vi "Write.vi"(8 "error in (no error)":errorcluster, 9 "timeout ms (5000)":i32=5000, 10 "Bytes to write":u8[](array[numeric]), 11 "dotNET SSL Socket in":refnum<class "dotNET SSL Socket.lvclass">) -> (0 "error out":errorcluster, 2 "bytes written":i32, 3 "dotNET SSL Socket out":refnum<class "dotNET SSL Socket.lvclass">)   [LabVIEW 2013, in "dotNET SSL Socket.lvlib" / "dotNET SSL Socket.lvclass"]
doc: "Writes data to the socket.\nWebSockets 2.0.0.30\nSam Sharp - MediaMongrels Ltd\nCopyright (c) 2019, MediaMongrels Ltd"
uses:
  dotNET SSL Socket.lvclass
  dotNET SSL Socket.lvclass/dotNET SSL Socket.ctl
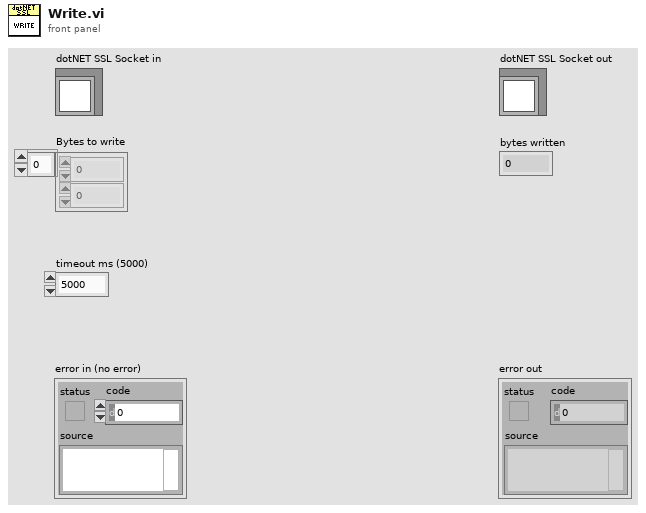
[diagram p1: front panel]
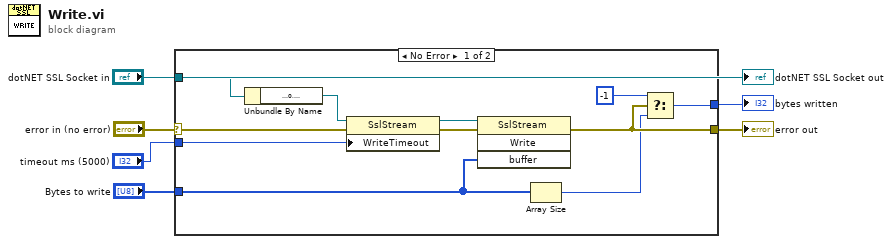
[diagram p0: block diagram]
diagram:
  n1 = case shown="No Error" "error in (no error)" {
    selector: "error in (no error)" -> [w7 w18]
    tunnel: "dotNET SSL Socket in" -> [w16 _]
    tunnel: "timeout ms (5000)" -> [w15 _]
    tunnel: [w12 w18] -> w4
    tunnel: [w11 _] -> w3
    tunnel: "Bytes to write" -> [w10 _]
    frame No Error {
      n2 = Unbundle By Name(w16) -> ("SSLStream"=w17:refnum<k24>)
      n3 = property class="SslStream"(reference=w17, error in=w7, "WriteTimeout"=w15) -> (reference out=w14:refnum<k24>, error out=w13:errorcluster)
      n4 = invoke class="SslStream" method="Write"(reference=w14, error in=w13, "buffer"=w10) -> (error out=w12:errorcluster)  [unwired: 1 in, 3 out]
      n5 = Array Size(array=w10) -> (size(s)=w9:i32)
      n6 = Select(t=-1, s=w12, f=w9) -> (s? t:f=w11:i32)
    }
    frame Error {
    }
  }
  "error out" <- w4
  "bytes written" <- w3
  "dotNET SSL Socket out" <- "dotNET SSL Socket in"
